vi "NextronTemperatureControl_v1.vi"() -> ()   [LabVIEW 2023]
uses:
  NXTStates.ctl
panel:
  in  "Ctrl":bool=TRUE
  in  "TPD":bool
  in  "Steps":cluster{"t (s)":dbl, "T (°C)":dbl}[](array[cluster]) {"T (°C)" min=-50.0 max=50.0 step=0.01}
  out "Temperature °C":dbl
  in  "Set Point (°C)":dbl=20.0 min=20.0 max=450.0 step=1.0
  out "Nextron Ramp Parameters":T1
  in  "Power":bool
  out "MSG/Err":string
  in  "Stop":bool
  out "Temperature":cluster{dbl[], dbl[]}[](graph)
  # "2o25, M. Hruska (hruskaa@vscht.cz)"
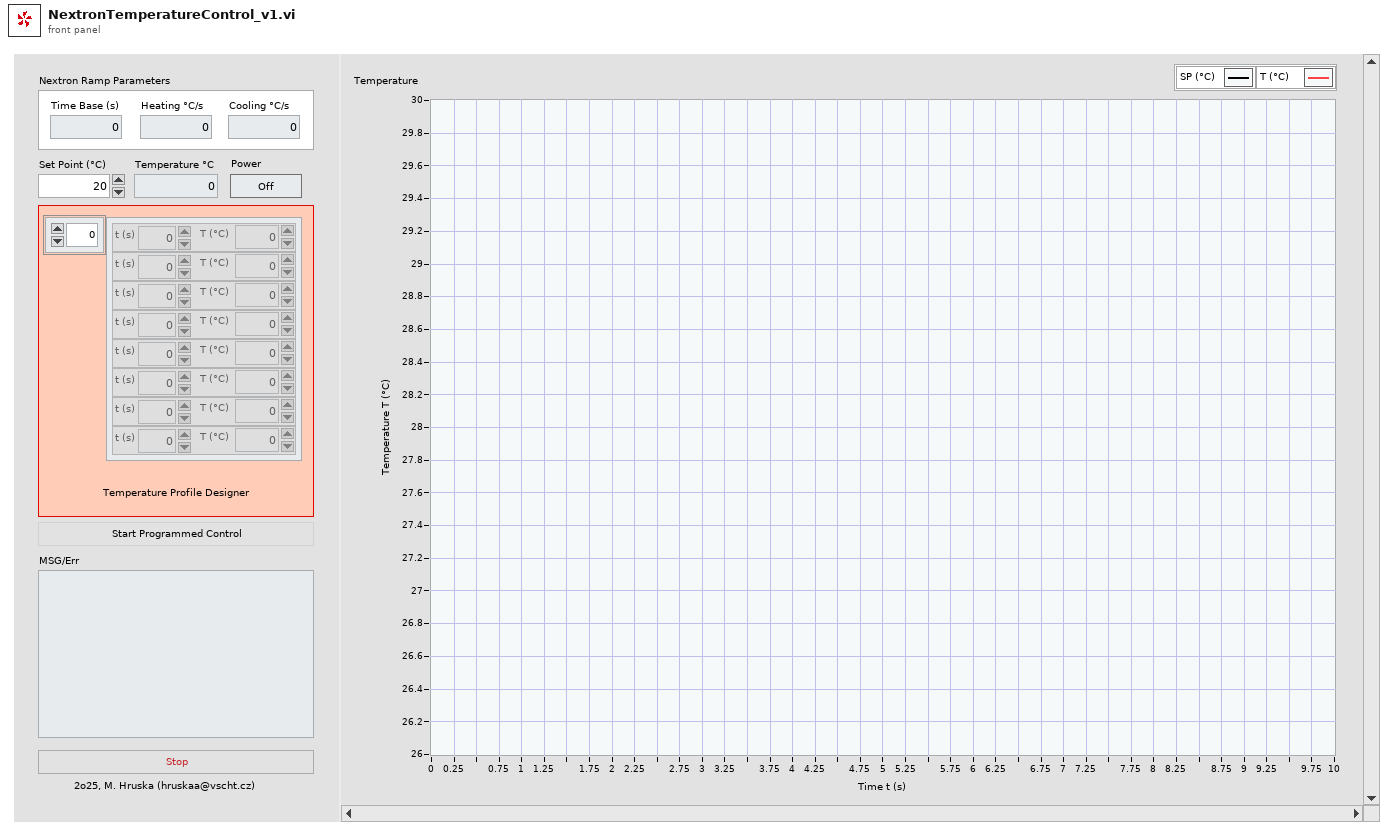
[diagram p1: front panel]
types:
  T1 = cluster{"Time Base (s)":dbl, "Heating °C/s":dbl, "Cooling °C/s":dbl}
  T2 = typedef "NXTStates.ctl" = enum16{"Init", "Manual", "Close", "Programmed"}
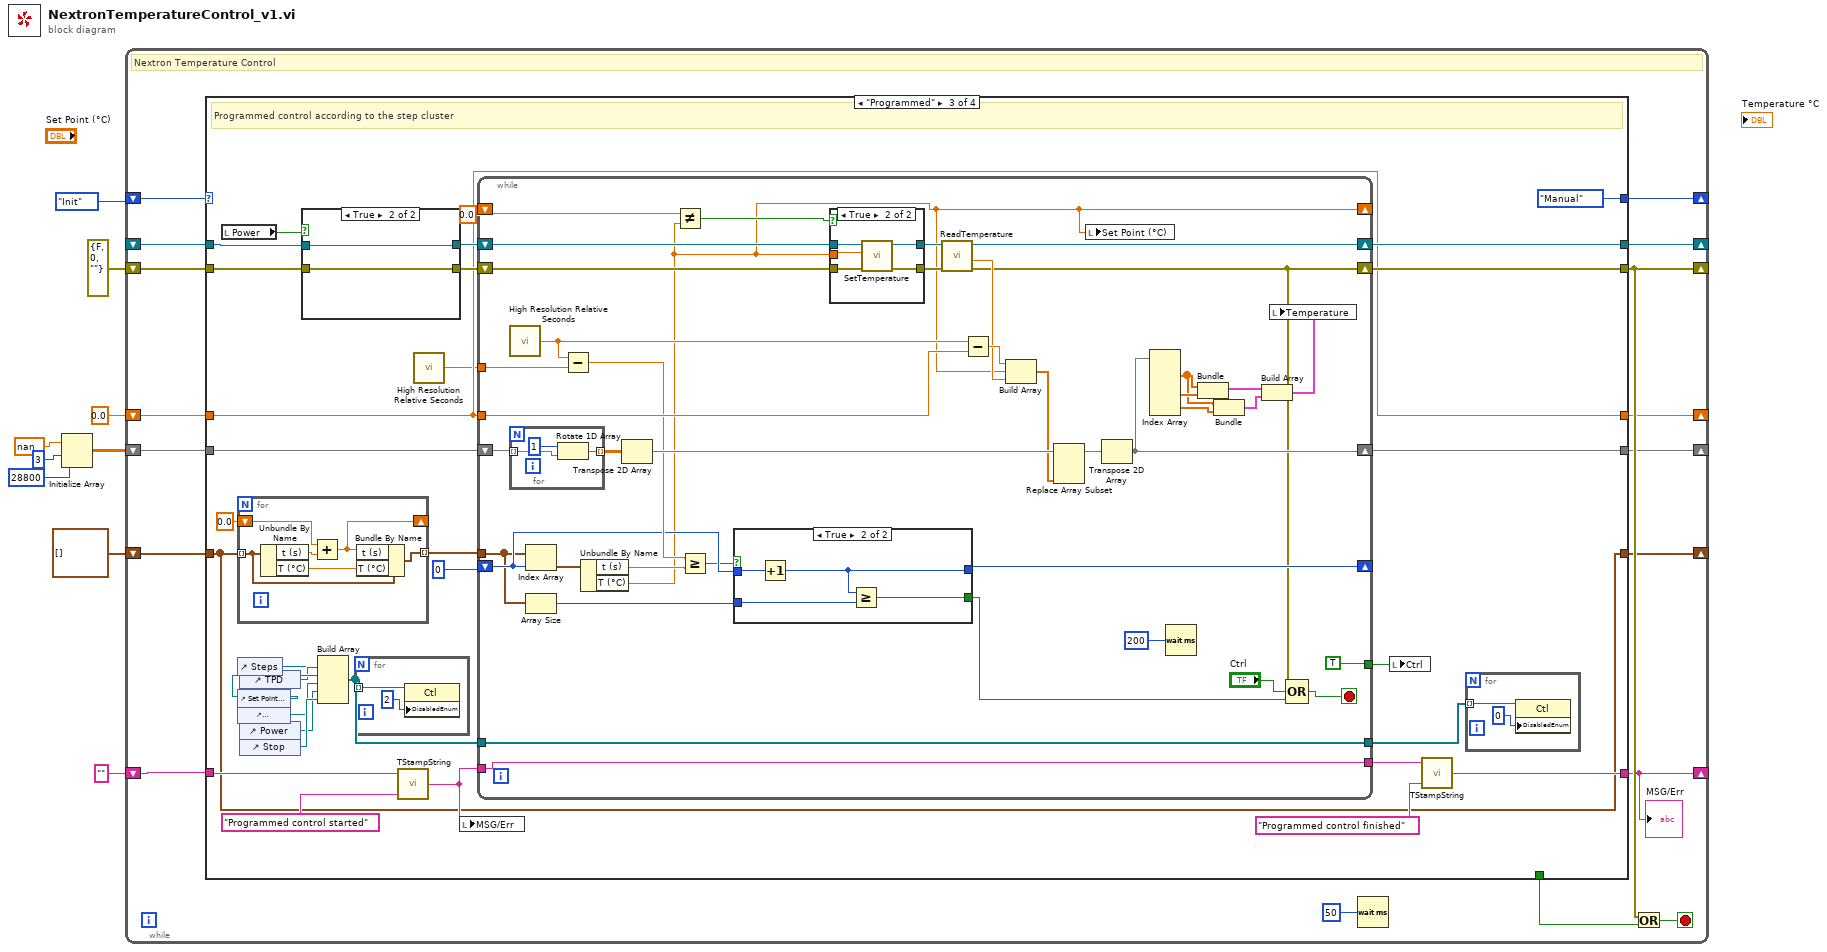
[diagram p0: block diagram]
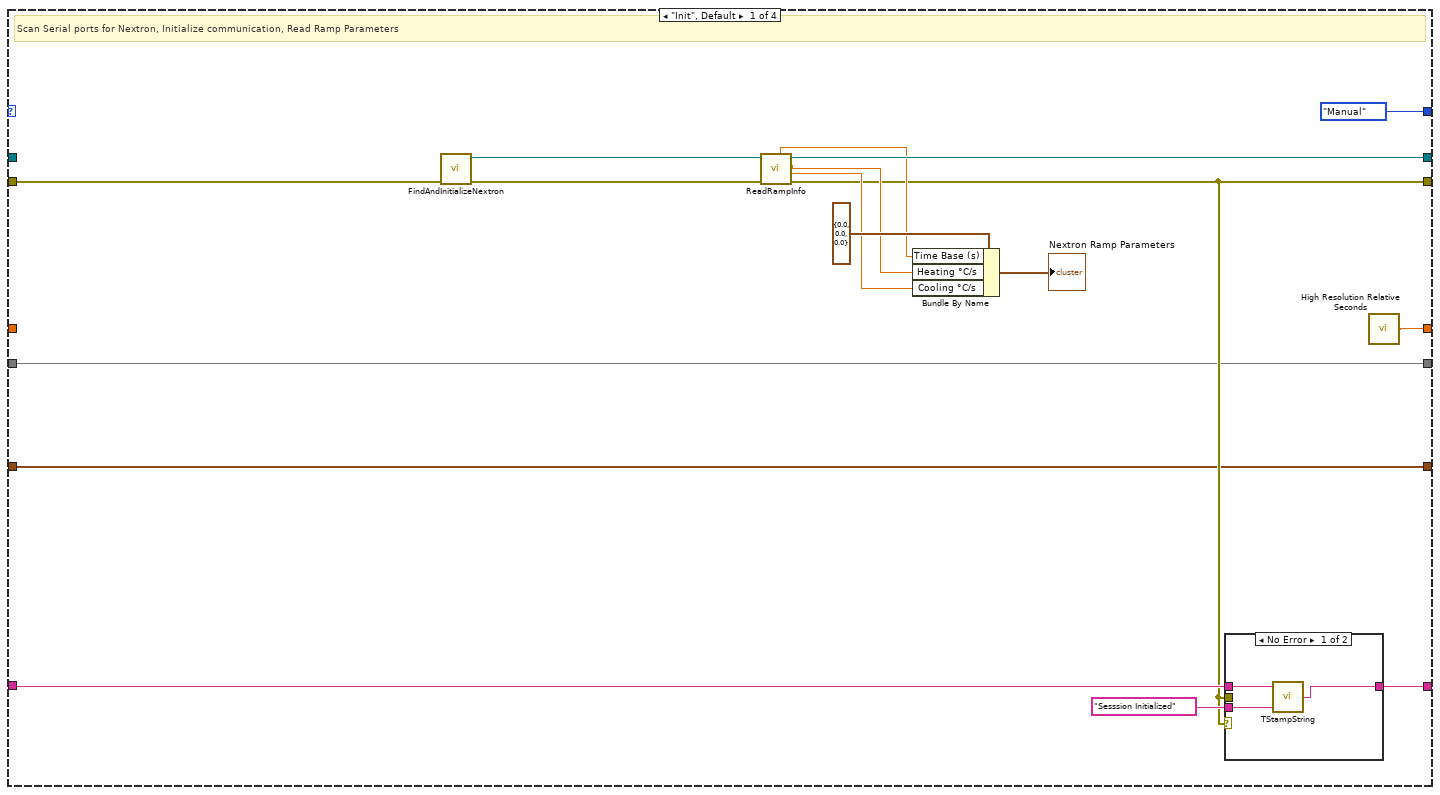
[diagram p2: hidden frame]
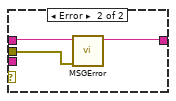
[diagram p3: hidden frame]
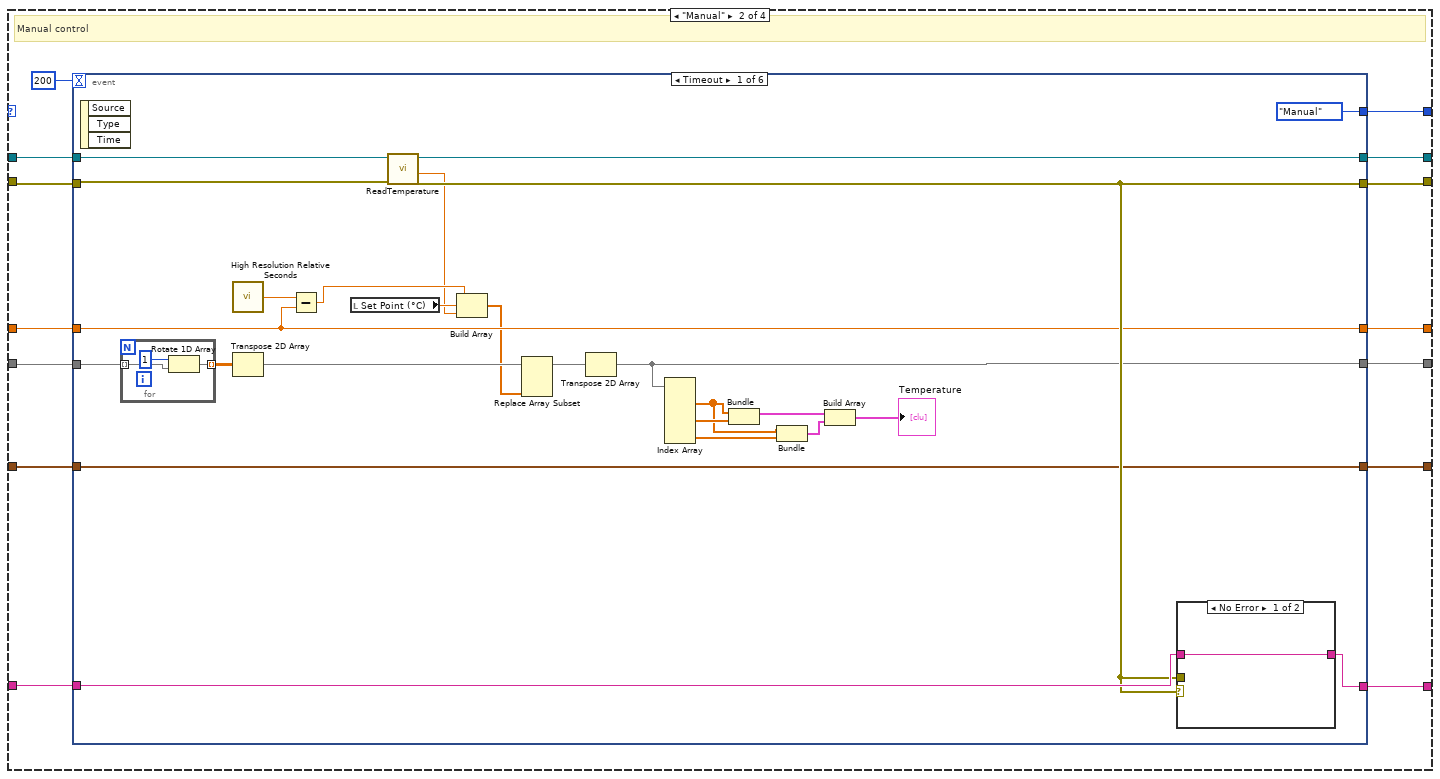
[diagram p4: hidden frame]
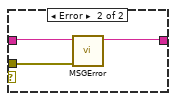
[diagram p5: hidden frame]
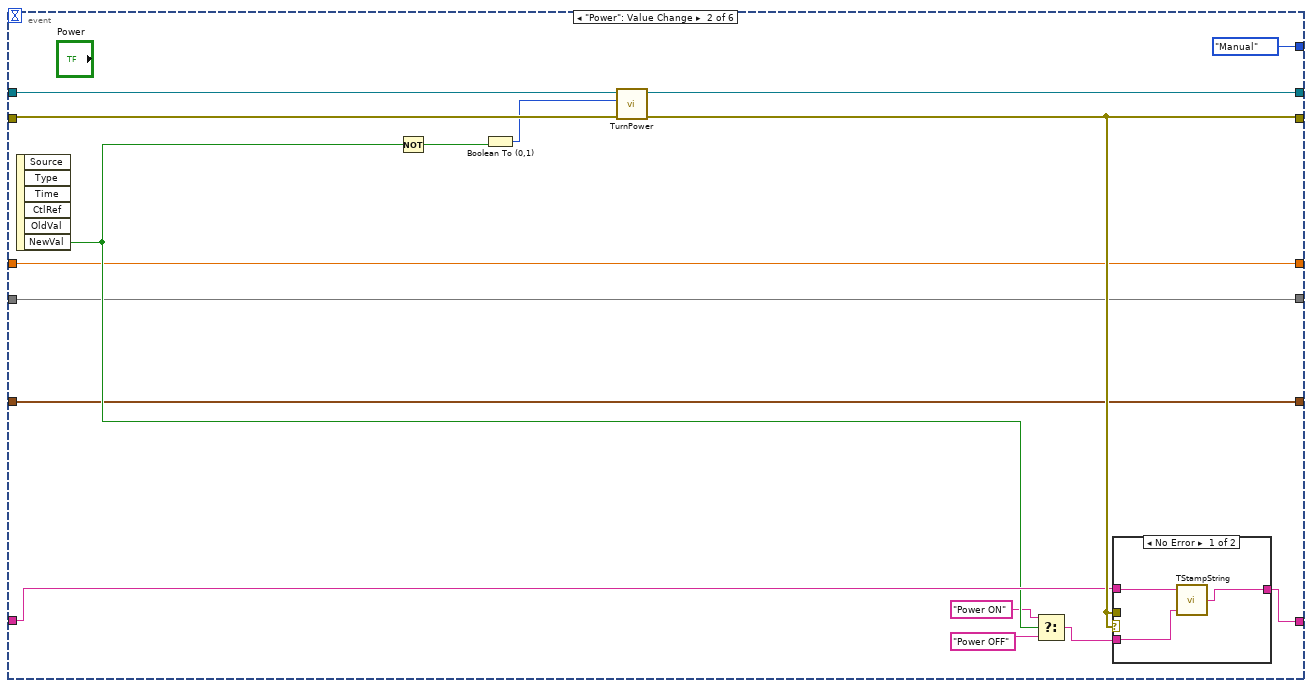
[diagram p6: hidden frame]
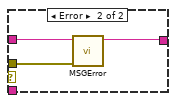
[diagram p7: hidden frame]
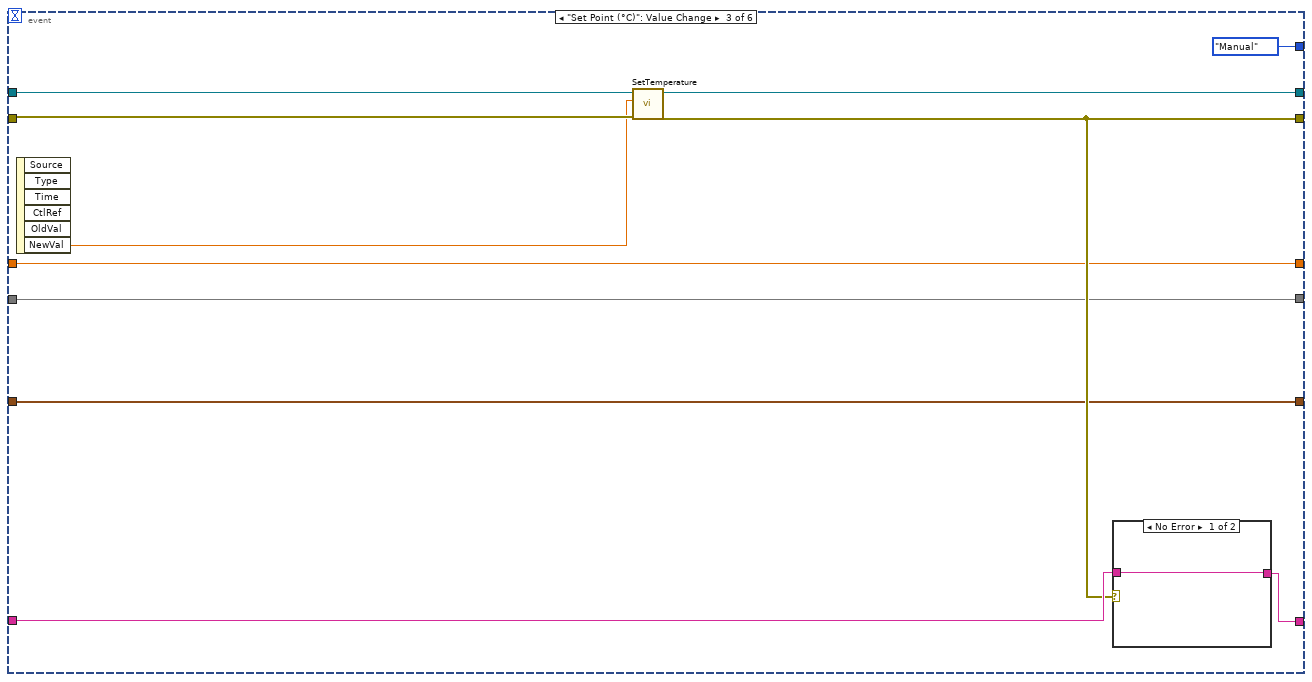
[diagram p8: hidden frame]
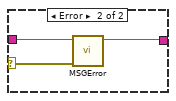
[diagram p9: hidden frame]
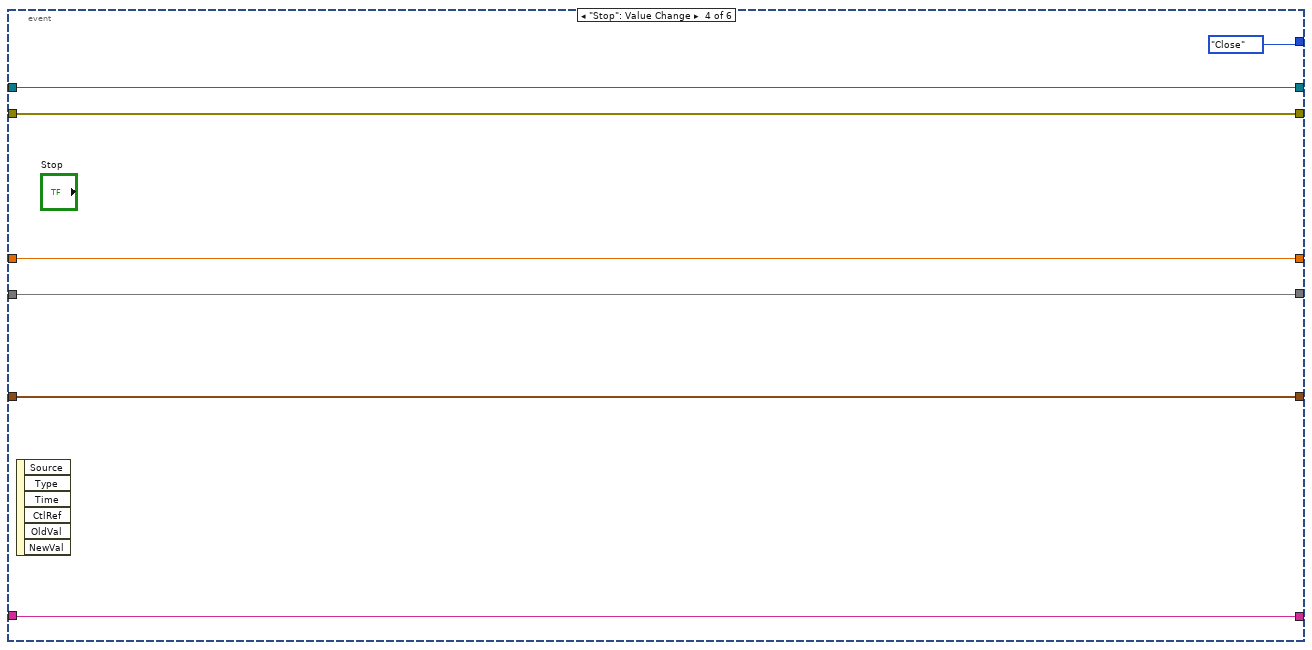
[diagram p10: hidden frame]
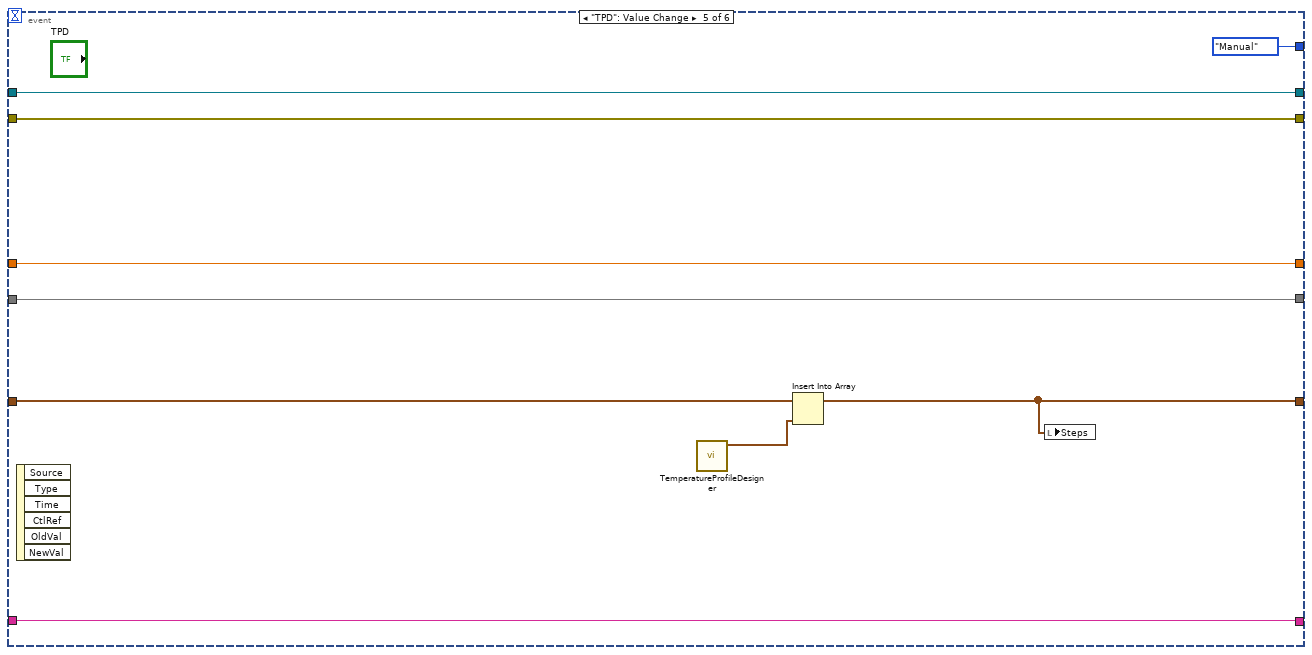
[diagram p11: hidden frame]
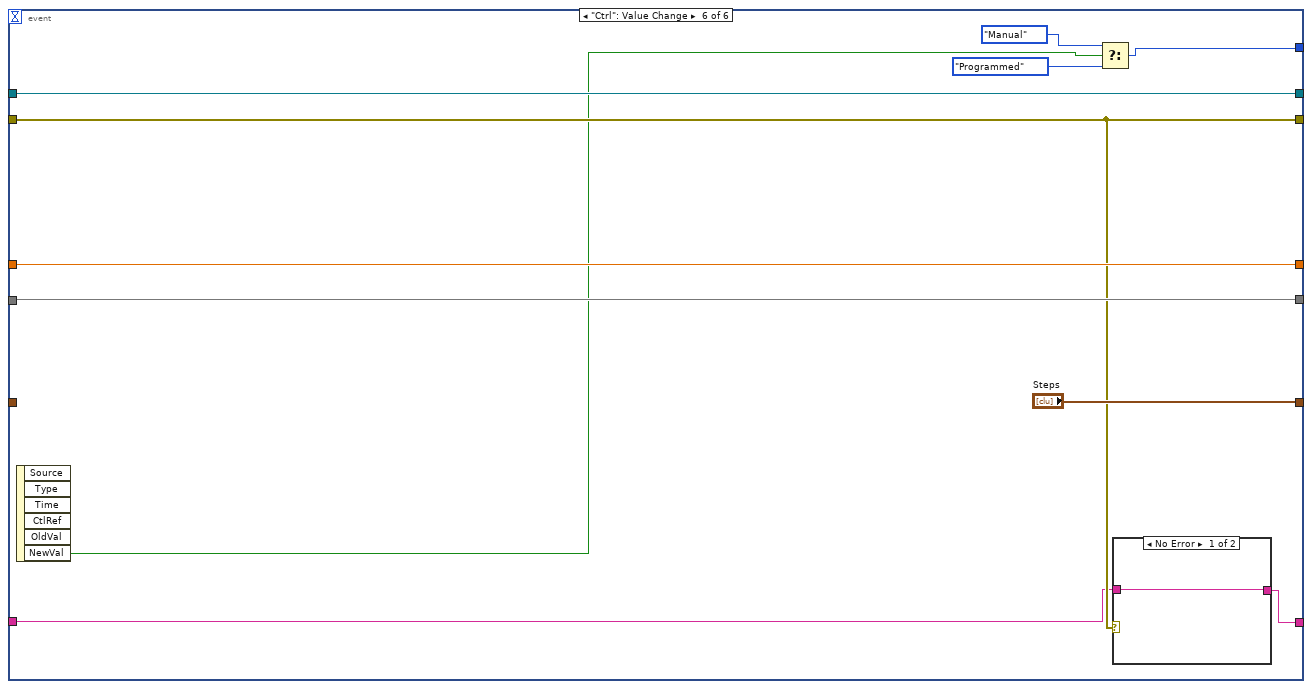
[diagram p12: hidden frame]
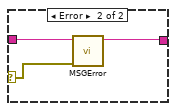
[diagram p13: hidden frame]
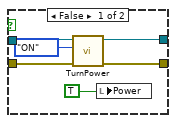
[diagram p14: hidden frame]
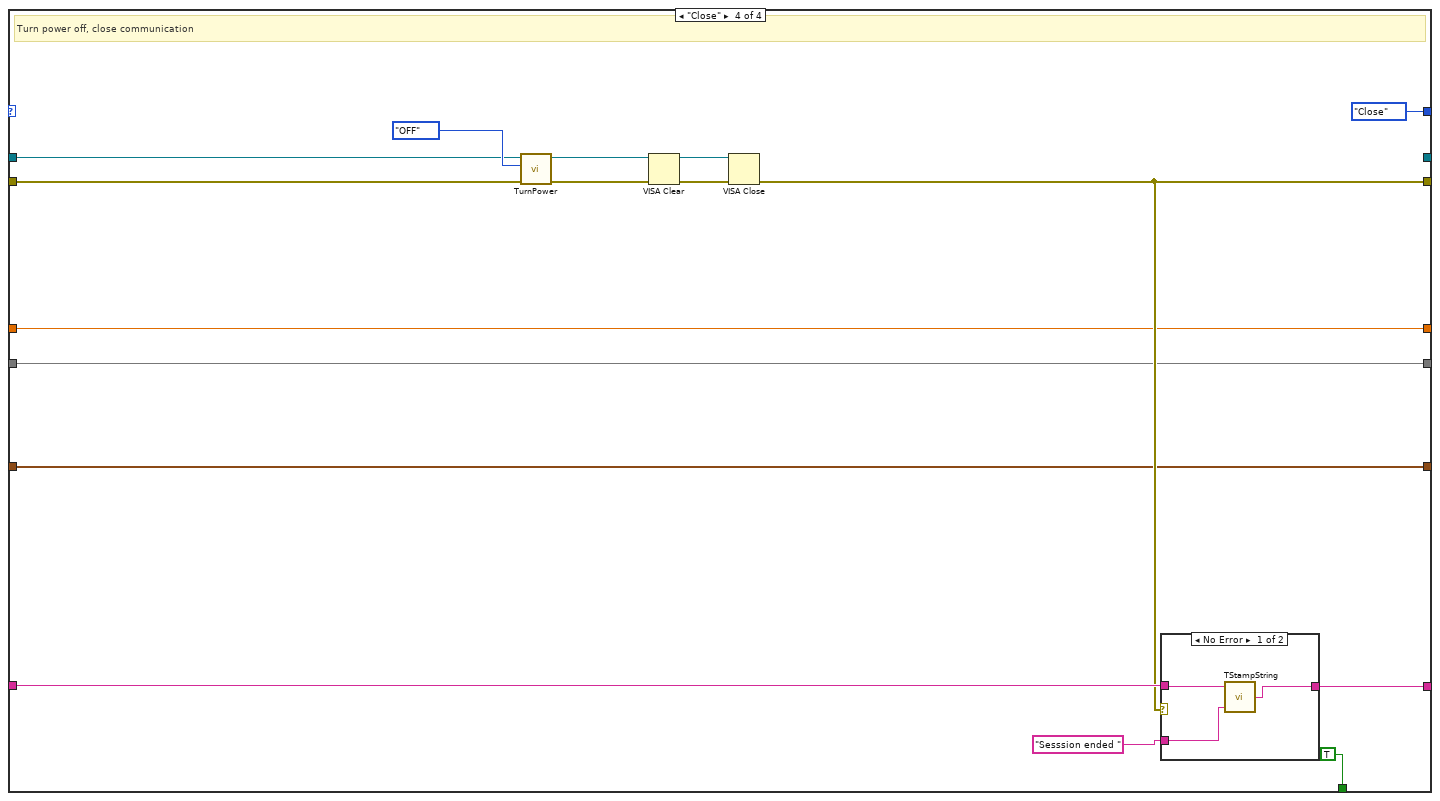
[diagram p17: hidden frame]
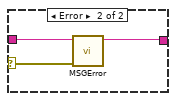
[diagram p18: hidden frame]
diagram:
  n1 = Initialize Array(nan ("element"), 3 ("dimension size"), 28800 ("dimension size")) -> (w6:dbl[][])
  n2 = while {
    shift-right: [w25] -> _
    shift-left: NXTStates."Init" -> [w26]
    shift-right: [w22] -> _
    shift-left: errorcluster {"status"=FALSE, "code"=0, "source"=""} ("error out") -> [w24]
    shift-right: [w20] -> _
    shift-left: _ -> [w19]
    shift-right: [w17] -> _
    shift-left: "" -> [w18]
    shift-right: [w12] -> _
    shift-left: w6 -> [w15]
    shift-right: [w14] -> _
    shift-left: 0.0 ("relative seconds") -> [w13]
    shift-right: [w10] -> _
    shift-left: cluster{"t (s)":dbl, "T (°C)":dbl}[] [] ("Steps") -> [w11]
    stop <- w23 stop-if-true
    # "Nextron Temperature Control"
    n3 = case shown="\"Programmed\"" w26 {
      tunnel: [NXTStates."Manual" w63 NXTStates."Manual" NXTStates."Close"] -> w25
      tunnel: [w30 w62 w188 w274] -> w22
      tunnel: w24 -> [w42 w61 w193 w284]
      tunnel: [_ _ _ TRUE] -> w21
      tunnel: [w40 w59 w189 _] -> w20
      tunnel: w19 -> [_ w60 w192 w282]
      tunnel: [w32 w56 w180 w276] -> w17
      tunnel: w18 -> [w33 w57 w184 w275]
      tunnel: w15 -> [w28 w53 w187 w271]
      tunnel: [w29 w54 w178 w272] -> w14
      tunnel: w13 -> [_ w55 w178 w272]
      tunnel: [w28 w52 w186 w271] -> w12
      tunnel: w11 -> [w27 w51 w175 w270]
      tunnel: [w27 w50 w175 w270] -> w10
      frame "Init", Default {
        # "Scan Serial ports for Nextron, Initialize communication, Read Ramp Parameters"
        n4 = call "FindAndInitializeNextron.vi"("error in (no error)"=w42) -> ("error in (no error) 2"=w41:errorcluster, "VISA Refnum Out"=w39:refnum<visa-resource-name>)  [unwired: 9 in]
        n5 = call "ReadRampInfo.vi"("error in (no error)"=w41, "VISA Refnum in"=w39) -> ("error in (no error) 2"=w30:errorcluster, "Cooling Ramp °C/s"=w34:dbl, "Heating Ramp °C/s"=w35:dbl, "VISA Refnum Out"=w40:refnum<visa-resource-name>, "Time base (s)"=w36:dbl)  [unwired: 5 in]
        n6 = Bundle By Name(cluster=T1 {"Time Base (s)"=0.0, "Heating °C/s"=0.0, "Cooling °C/s"=0.0} ("Nextron Ramp Parameters"), "Time Base (s)"=w36, "Heating °C/s"=w35, "Cooling °C/s"=w34) -> (→"Nextron Ramp Parameters":T1)
        n7 = case shown="No Error" w30 {
          tunnel: w33 -> [w46 w49]
          tunnel: [w45 w48] -> w32
          tunnel: "Sesssion Initialized" -> [w44 _]
          tunnel: w30 -> [_ w47]
          frame No Error {
            n8 = call "TStampString.vi"("Incoming string"=w44, "Previous string"=w46) -> ("String with time stamp"=w45:string)  [unwired: 1 in]
          }
          frame Error {
            n9 = call "MSGError.vi"("error in (no error)"=w47, "IncomingString"=w49) -> ("OutputString"=w48:string)  [unwired: 8 in, 1 out]
          }
        }
        n10 = call <vilib>:"High Resolution Relative Seconds.vi"() -> ("relative seconds"=w29:dbl)
      }
      frame "Manual" {
        # "Manual control"
        n11 = event shown="[0] Timeout" {
          selector: _ -> [_ _ _ _ _ _]
          dyn-events: _ -> [_ _ _ _ _ _]
          timeout: 200 -> [_ _ _ _ _ _]
          tunnel: [NXTStates."Manual" NXTStates."Manual" NXTStates."Manual" NXTStates."Close" NXTStates."Manual" w150] -> w63
          tunnel: [w82 w104 w121 w137 w148 w154] -> w62
          tunnel: w61 -> [w88 w111 w128 w137 w148 w154]
          tunnel: w60 -> [w87 w108 w127 w138 w147 w159]
          tunnel: [w86 w107 w126 w138 w147 w159] -> w59
          tunnel: w57 -> [w83 w103 w122 w136 w140 w153]
          tunnel: [w84 w105 w123 w136 w140 w155] -> w56
          tunnel: w55 -> [w80 w98 w120 w135 w145 w158]
          tunnel: [w80 w98 w120 w135 w145 w158] -> w54
          tunnel: w53 -> [w79 w97 w119 w134 w144 w157]
          tunnel: [w71 w97 w119 w134 w144 w157] -> w52
          tunnel: w51 -> [w64 w96 w118 w133 w143 _]
          tunnel: [w64 w96 w118 w133 w141 "Steps"] -> w50
          event Timeout {
            n12 = event-data() -> ()  [unwired: 1 in, 3 out]
            n13 = for {
              tunnel: [w90] -> w78 mode=indexing
              tunnel: w79 -> [w89] mode=indexing
              n14 = Rotate 1D Array(1:w89, 2:1 ("n")) -> (0:w90:dbl[])
            }
            n15 = call <vilib>:"High Resolution Relative Seconds.vi"() -> ("relative seconds"=w81:dbl)
            n16 = Transpose 2D Array(2D array=w78) -> (transposed array=w77:dbl[][])
            n17 = Subtract(x=w81, y=w80) -> (x-y=w75:dbl)
            n18 = local read "Set Point (°C)"() -> (w74:dbl)
            n19 = call "ReadTemperature.vi"("error in (no error)"=w88, "VISA Refnum in"=w87) -> ("error in (no error) 2"=w82:errorcluster, "Temperature (°C)"=w73:dbl, "VISA Refnum Out"=w86:refnum<visa-resource-name>)  [unwired: 6 in, 1 out]
            n20 = Build Array(w75, w74, w73) -> (w72:dbl[])
            n21 = Replace Array Subset(array=w77, new element=w72) -> (w76:dbl[][])  [unwired: 2 in]
            n22 = Transpose 2D Array(2D array=w76) -> (transposed array=w71:dbl[][])
            n23 = Index Array(array=w71) -> (element #1=w69:dbl[], element #2=w70:dbl[], element #3=w68:dbl[])  [unwired: 6 in]
            n24 = Bundle(w69, w70) -> (w67:cluster{dbl[], dbl[]})  [unwired: 1 in]
            n25 = Bundle(w69, w68) -> (w66:cluster{dbl[], dbl[]})  [unwired: 1 in]
            n26 = Build Array(w67, w66) -> (→"Temperature":cluster{dbl[], dbl[]}[])
            n27 = case shown="No Error" w82 {
              tunnel: w83 -> [w92 w95]
              tunnel: [w92 w94] -> w84
              tunnel: w82 -> [_ w93]
              frame No Error {
              }
              frame Error {
                n28 = call "MSGError.vi"("error in (no error)"=w93, "IncomingString"=w95) -> ("OutputString"=w94:string)  [unwired: 8 in, 1 out]
              }
            }
          }
          event "Power": Value Change {
            n29 = event-data() -> ("NewVal"=w101:bool)  [unwired: 1 in, 5 out]
            n30 = Not(x=w101) -> (.not. x?=w110:bool)
            n31 = Boolean To (0,1)(Boolean=w110) -> (0, 1=w109:i16)
            n32 = call "TurnPower.vi"("error in (no error)"=w111, "Power ON/OFF"=w109, "VISA Refnum in"=w108) -> ("error in (no error) 2"=w104:errorcluster, "VISA Refnum Out"=w107:refnum<visa-resource-name>)  [unwired: 7 in]
            n33 = Select(t="Power ON", s=w101, f="Power OFF") -> (s? t:f=w102:string)
            n34 = case shown="No Error" w104 {
              tunnel: [w113 w117] -> w105
              tunnel: w104 -> [_ w116]
              tunnel: w103 -> [w114 w115]
              tunnel: w102 -> [w112 _]
              frame No Error {
                n35 = call "TStampString.vi"("Incoming string"=w112, "Previous string"=w114) -> ("String with time stamp"=w113:string)  [unwired: 1 in]
              }
              frame Error {
                n36 = call "MSGError.vi"("error in (no error)"=w116, "IncomingString"=w115) -> ("OutputString"=w117:string)  [unwired: 8 in, 1 out]
              }
            }
          }
          event "Set Point (°C)": Value Change {
            n37 = event-data() -> ("NewVal"=w125:dbl)  [unwired: 1 in, 5 out]
            n38 = call "SetTemperature.vi"("error in (no error)"=w128, "Temperature (°C)"=w125, "VISA Refnum in"=w127) -> ("error in (no error) 2"=w121:errorcluster, "VISA Refnum Out"=w126:refnum<visa-resource-name>)  [unwired: 7 in]
            n39 = case shown="No Error" w121 {
              selector: w121 -> [_ w130]
              tunnel: [w129 w132] -> w123
              tunnel: w122 -> [w129 w131]
              frame No Error {
              }
              frame Error {
                n40 = call "MSGError.vi"("error in (no error)"=w130, "IncomingString"=w131) -> ("OutputString"=w132:string)  [unwired: 8 in, 1 out]
              }
            }
          }
          event "Stop": Value Change {
            n41 = event-data() -> ()  [unwired: 1 in, 6 out]
          }
          event "TPD": Value Change {
            n42 = event-data() -> ()  [unwired: 1 in, 6 out]
            n43 = call "TemperatureProfileDesigner.vi"() -> ("ShcemeCluster"=w142:cluster{"Time":dbl, "Voltage":dbl}[])  [unwired: 11 in]
            n44 = Insert Into Array(array=w143, new element=w142) -> (w141:cluster{"t (s)":dbl, "T (°C)":dbl}[])  [unwired: 1 in]
            n45 = local write "Steps"(w141) -> ()
          }
          event "Ctrl": Value Change {
            n46 = event-data() -> ("NewVal"=w149:bool)  [unwired: 1 in, 5 out]
            n47 = Select(t=NXTStates."Manual", s=w149, f=NXTStates."Programmed") -> (s? t:f=w150:T2)
            n48 = case shown="No Error" w154 {
              selector: w154 -> [_ w161]
              tunnel: [w160 w163] -> w155
              tunnel: w153 -> [w160 w162]
              frame No Error {
              }
              frame Error {
                n49 = call "MSGError.vi"("error in (no error)"=w161, "IncomingString"=w162) -> ("OutputString"=w163:string)  [unwired: 8 in, 1 out]
              }
            }
          }
        }
      }
      frame "Programmed" {
        # "Programmed control according to the step cluster"
        n50 = local read "Power"() -> (w194:bool)
        n51 = for {
          tunnel: w175 -> [w203] mode=indexing
          shift-right: [w201] -> _
          shift-left: 0.0 -> [w204]
          tunnel: [w202] -> w173 mode=indexing
          n52 = Unbundle By Name(w203) -> ("t (s)"=w205:dbl, "T (°C)"=w200:dbl)
          n53 = Add(x=w204, y=w205) -> (x+y=w201:dbl)
          n54 = Bundle By Name(cluster=w203, "t (s)"=w201, "T (°C)"=w200) -> (w202:cluster{"t (s)":dbl, "T (°C)":dbl})
        }
        n55 = control-ref of="Steps"() -> (w166:refnum<vi>)
        n56 = control-ref of="Set Point (°C)"() -> (w168:refnum<vi>)
        n57 = control-ref of="Temperature °C"() -> (w169:refnum<vi>)
        n58 = control-ref of="TPD"() -> (w167:refnum<vi>)
        n59 = control-ref of="Power"() -> (w170:refnum<vi>)
        n60 = control-ref of="Stop"() -> (w171:refnum<vi>)
        n61 = case shown="True" w194 {
          tunnel: w193 -> [w211 w212]
          tunnel: w192 -> [w210 w213]
          tunnel: [w207 w213] -> w191
          tunnel: [w206 w212] -> w190
          frame False {
            n62 = call "TurnPower.vi"("error in (no error)"=w211, "Power ON/OFF"=enum16{"ON", "OFF"}."ON", "VISA Refnum in"=w210) -> ("error in (no error) 2"=w206:errorcluster, "VISA Refnum Out"=w207:refnum<visa-resource-name>)  [unwired: 7 in]
            n63 = local write "Power"(TRUE ("Power")) -> ()
          }
          frame True {
          }
        }
        n64 = Build Array(w166, w167, w168, w169, w170, w171) -> (w165:refnum<vi>[])
        n65 = for {
          tunnel: w165 -> [w199] mode=indexing
          n66 = property class="Ctl"(reference=w199, "DisabledEnum"=2) -> ()  [unwired: 1 in, 2 out]
        }
        n67 = call "TStampString.vi"("Incoming string"="Programmed control started", "Previous string"=w184) -> ("String with time stamp"=w182:string)  [unwired: 1 in]
        n68 = call <vilib>:"High Resolution Relative Seconds.vi"() -> ("relative seconds"=w177:dbl)
        n69 = local write "MSG/Err"(w182) -> ()
        n70 = while {
          shift-right: [w250] -> w189
          shift-left: w191 -> [w254]
          shift-right: [w219] -> w188
          shift-left: w190 -> [w253]
          shift-right: [w241] -> w186
          shift-left: w187 -> [w247]
          tunnel: w178 -> [w244]
          tunnel: [TRUE] -> w185
          tunnel: w182 -> [w248]
          tunnel: [w248] -> w181
          tunnel: w173 -> [w221]
          tunnel: w177 -> [w230]
          shift-right: [w225] -> _
          shift-left: 0 -> [w226]
          shift-right: [w215] -> _
          shift-left: 0.0 -> [w223]
          tunnel: w165 -> [w214]
          tunnel: [w214] -> w164
          stop <- w218 stop-if-true
          n71 = call <vilib>:"High Resolution Relative Seconds.vi"() -> ("relative seconds"=w231:dbl)
          n72 = for {
            tunnel: [w268] -> w246 mode=indexing
            tunnel: w247 -> [w267] mode=indexing
            n73 = Rotate 1D Array(1:w267, 2:1 ("n")) -> (0:w268:dbl[])
          }
          n74 = Index Array(array=w221, index=w226) -> (element=w229:cluster{"t (s)":dbl, "T (°C)":dbl})
          n75 = Array Size(array=w221) -> (size(s)=w220:i32)
          n76 = Subtract(x=w231, y=w230) -> (x-y=w227:dbl)
          n77 = Unbundle By Name(w229) -> ("t (s)"=w228:dbl, "T (°C)"=w215:dbl)
          n78 = Transpose 2D Array(2D array=w246) -> (transposed array=w243:dbl[][])
          n79 = Not Equal?(x=w223, y=w215) -> (x != y?=w222:bool)
          n80 = Greater Or Equal?(x=w227, y=w228) -> (x >= y?=w224:bool)
          n81 = case shown="True" w224 {
            tunnel: w226 -> [w255 w259]
            tunnel: [w255 w258] -> w225
            tunnel: w220 -> [_ w257]
            tunnel: [_ w256] -> w216
            frame False {
            }
            frame True {
              n82 = Increment(x=w259) -> (x+1=w258:i32)
              n83 = Greater Or Equal?(x=w258, y=w257) -> (x >= y?=w256:bool)
            }
          }
          n84 = case shown="True" w222 {
            tunnel: w254 -> [w261 w266]
            tunnel: w253 -> [w260 w265]
            tunnel: [w261 w264] -> w252
            tunnel: [w260 w263] -> w251
            tunnel: w215 -> [_ w262]
            frame False {
            }
            frame True {
              n85 = call "SetTemperature.vi"("error in (no error)"=w265, "Temperature (°C)"=w262, "VISA Refnum in"=w266) -> ("error in (no error) 2"=w263:errorcluster, "VISA Refnum Out"=w264:refnum<visa-resource-name>)  [unwired: 7 in]
            }
          }
          n86 = call "ReadTemperature.vi"("error in (no error)"=w251, "VISA Refnum in"=w252) -> ("error in (no error) 2"=w219:errorcluster, "Temperature (°C)"=w233:dbl, "VISA Refnum Out"=w250:refnum<visa-resource-name>)  [unwired: 6 in, 1 out]
          n87 = Subtract(x=w231, y=w244) -> (x-y=w245:dbl)
          n88 = Build Array(w245, w215, w233) -> (w234:dbl[])
          n89 = Replace Array Subset(array=w243, new element=w234) -> (w242:dbl[][])  [unwired: 2 in]
          n90 = local write "Set Point (°C)"(w215) -> ()
          n91 = Transpose 2D Array(2D array=w242) -> (transposed array=w241:dbl[][])
          n92 = Index Array(array=w241) -> (element #1=w239:dbl[], element #2=w240:dbl[], element #3=w238:dbl[])  [unwired: 6 in]
          n93 = Wait (ms)(milliseconds to wait=u32 200) -> ()  [unwired: 1 out]
          n94 = Bundle(w239, w240) -> (w237:cluster{dbl[], dbl[]})  [unwired: 1 in]
          n95 = Bundle(w239, w238) -> (w236:cluster{dbl[], dbl[]})  [unwired: 1 in]
          n96 = Build Array(w237, w236) -> (w235:cluster{dbl[], dbl[]}[])
          n97 = local write "Temperature"(w235) -> ()
          n98 = Compound Arithmetic op=OR(w219, "Ctrl", w216) -> (w218:bool)
        }
        n99 = local write "Ctrl"(w185) -> ()
        n100 = call "TStampString.vi"("Incoming string"="Programmed control finished", "Previous string"=w181) -> ("String with time stamp"=w180:string)  [unwired: 1 in]
        n101 = for {
          tunnel: w164 -> [w197] mode=indexing
          n102 = property class="Ctl"(reference=w197, "DisabledEnum"=0) -> ()  [unwired: 1 in, 2 out]
        }
      }
      frame "Close" {
        # "Turn power off, close communication"
        n103 = call "TurnPower.vi"("error in (no error)"=w284, "Power ON/OFF"=enum16{"ON", "OFF"}."OFF", "VISA Refnum in"=w282) -> ("error in (no error) 2"=w281:errorcluster, "VISA Refnum Out"=w280:refnum<visa-resource-name>)  [unwired: 7 in]
        n104 = VISA Clear(VISA resource name=w280, error in (no error)=w281) -> (VISA resource name out=w278:refnum<visa-resource-name>, error out=w279:errorcluster)
        n105 = VISA Close(VISA resource name=w278, error in (no error)=w279) -> (error out=w274:errorcluster)
        n106 = case shown="No Error" w274 {
          selector: w274 -> [_ w289]
          tunnel: [w287 w291] -> w276
          tunnel: w275 -> [w288 w290]
          tunnel: "Sesssion ended " -> [w286 _]
          frame No Error {
            n107 = call "TStampString.vi"("Incoming string"=w286, "Previous string"=w288) -> ("String with time stamp"=w287:string)  [unwired: 1 in]
          }
          frame Error {
            n108 = call "MSGError.vi"("error in (no error)"=w289, "IncomingString"=w290) -> ("OutputString"=w291:string)  [unwired: 8 in, 1 out]
          }
        }
      }
    }
    "MSG/Err" <- w17
    n109 = Wait (ms)(milliseconds to wait=u32 50) -> ()  [unwired: 1 out]
    n110 = Or(x=w22, y=w21) -> (x .or. y?=w23:bool)
  }
